vi "getClassInfo.vi"(0 "reference":refnum<class "ClassNode.lvclass">, 5 "error in (no error)":errorcluster) -> (9 "ClassPathUnmodified":path, 11 "methods(string)":string, 12 "Base class.bounds":T1 {"height" format="%.2f"; "width" format="%.2f"; "y" format="%.2f"; "x" format="%.2f"}, 13 "attributes(string)":string, 14 "reference out":refnum<class "ClassNode.lvclass">, 15 "className":string, 16 "attributes":string[](array[string]), 17 "methods":string[](array[string]), 18 "ClassPath":path, 19 "error out":errorcluster)   [LabVIEW 2012, in "ClassNode.lvclass"]
uses:
  <resource>/Framework/Providers/Open_GDS/UML/ClassNode_class/ClassNode.lvclass
  <resource>/Framework/Providers/Open_GDS/UML/General/Rectangle/Rectangle Rectangle2D.ctl
  <resource>/Framework/Providers/Open_GDS/UML/MultiLineString_class/MultiLineString.lvclass
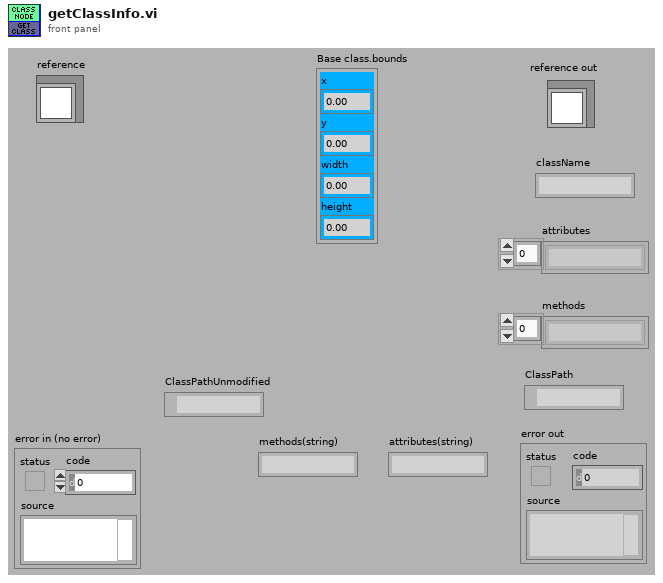
[diagram p1: front panel]
types:
  T1 = typedef "Rectangle Rectangle2D.ctl" = cluster{"x":dbl, "y":dbl, "width":dbl, "height":dbl}
  T2 = typedef "ClassNode.lvclass/ObjectAttributes.ctl" = cluster{"Base class":T3, "midHeight":dbl, "botHeight":dbl, "name":refnum<class "MultiLineString.lvclass">, "attributes":refnum<class "MultiLineString.lvclass">, "methods":refnum<class "MultiLineString.lvclass">, "DEFAULT_COMPARTMENT_HEIGHT":i32, "DEFAULT_WIDTH":i32, "DEFAULT_HEIGHT":i32, "showMethods":bool, "showAttributes":bool, "ClassPath":path}
  T3 = typedef "RectangularNode.lvclass/ObjectAttributes.ctl" = cluster{"Base class":T4, "bounds":T1}
  T4 = typedef "AbstractNode.lvclass/ObjectAttributes.ctl" = cluster{"parent":refnum<class "AbstractNode.lvclass">, "children":refnum<class "AbstractNode.lvclass">[], "Hidden":bool}
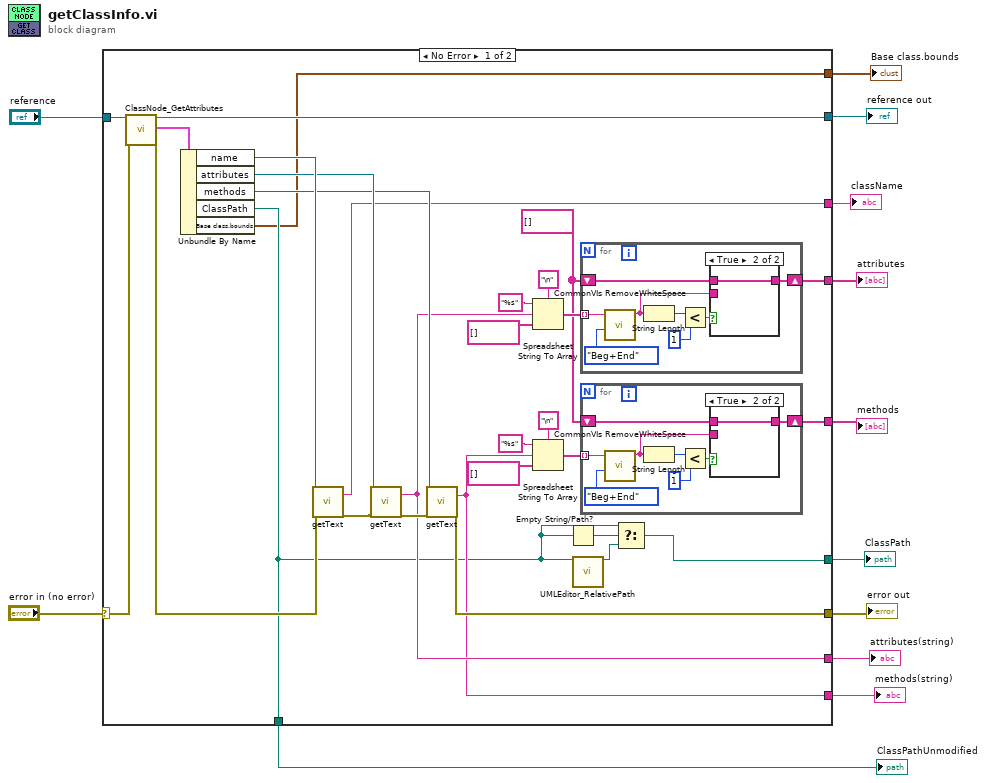
[diagram p0: block diagram]
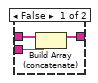
[diagram p2: hidden frame]
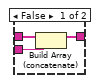
[diagram p3: hidden frame]
diagram:
  n1 = case shown="No Error" "error in (no error)" {
    selector: "error in (no error)" -> [w42 w67]
    tunnel: "reference" -> [w41 w68]
    tunnel: [w35 w67] -> w10
    tunnel: [w39 w68] -> w9
    tunnel: [w31 _] -> w8
    tunnel: [w26 _] -> w7
    tunnel: [w21 _] -> w6
    tunnel: [w14 _] -> w5
    tunnel: [w19 _] -> w4
    tunnel: [w18 _] -> w3
    tunnel: [w16 _] -> w2
    tunnel: [w13 _] -> w1
    frame No Error {
      w20 = string[] []
      n2 = call <resource>:"ClassNode_GetAttributes.vi"("reference in"=w41, "error in (no error)"=w42) -> ("reference out"=w39:refnum<class "ClassNode.lvclass">, "Attributes"=w40:T2, "error out"=w38:errorcluster)  [unwired: 15 out]
      n3 = Unbundle By Name(w40) -> ("name"=w34:refnum<class "MultiLineString.lvclass">, "attributes"=w33:refnum<class "MultiLineString.lvclass">, "methods"=w32:refnum<class "MultiLineString.lvclass">, "ClassPath"=w16:path, "Base class.bounds"=w13:T1)
      n4 = call-dynamic "getText.vi"("reference"=w34, "error in (no error)"=w38) -> ("text"=w31:string, "error out"=w37:errorcluster)  [unwired: 16 out]
      n5 = call-dynamic "getText.vi"("reference"=w33, "error in (no error)"=w37) -> ("text"=w19:string, "error out"=w36:errorcluster)  [unwired: 16 out]
      n6 = call-dynamic "getText.vi"("reference"=w32, "error in (no error)"=w36) -> ("text"=w18:string, "error out"=w35:errorcluster)  [unwired: 16 out]
      n7 = Spreadsheet String To Array(delimiter (Tab)="\n", format string="%s", spreadsheet string=w19, array type (2D Dbl)=string[] []) -> (array=w27:string[])
      n8 = Spreadsheet String To Array(delimiter (Tab)="\n", format string="%s", spreadsheet string=w18, array type (2D Dbl)=string[] []) -> (array=w25:string[])
      n9 = Empty String/Path?(string/path=w16) -> (empty?=w17:bool)
      n10 = call <resource>:"UMLEditor_RelativePath.vi"("Path In"=w16) -> ("ConvertToAbsolutePath(If possible)"=w15:path)  [unwired: 1 in, 17 out]
      n11 = for {
        tunnel: w27 -> [w62] mode=indexing
        shift-right: [w55] -> w26
        shift-left: w20 -> [w57]
        n12 = call <resource>:"CommonVIs RemoveWhiteSpace.vi"("Remove from"=enum16{"Begining", "End", "Beg+End", "All"}."Beg+End", "String in"=w62) -> ("String out"=w56:string)  [unwired: 2 in, 3 out]
        n13 = String Length(string=w56) -> (length=w60:i32)
        n14 = Less?(x=w60, y=1) -> (x < y?=w58:bool)
        n15 = case shown="True" w58 {
          tunnel: w57 -> [w65 w66]
          tunnel: w56 -> [w64 _]
          tunnel: [w63 w66] -> w55
          frame False {
            n16 = Build Array (concatenate)(w65, w64) -> (w63:string[])
          }
          frame True {
          }
        }
      }
      n17 = for {
        tunnel: w25 -> [w50] mode=indexing
        shift-right: [w43] -> w21
        shift-left: w20 -> [w45]
        n18 = call <resource>:"CommonVIs RemoveWhiteSpace.vi"("Remove from"=enum16{"Begining", "End", "Beg+End", "All"}."Beg+End", "String in"=w50) -> ("String out"=w44:string)  [unwired: 2 in, 3 out]
        n19 = String Length(string=w44) -> (length=w48:i32)
        n20 = Less?(x=w48, y=1) -> (x < y?=w46:bool)
        n21 = case shown="True" w46 {
          tunnel: w45 -> [w53 w54]
          tunnel: w44 -> [w52 _]
          tunnel: [w51 w54] -> w43
          frame False {
            n22 = Build Array (concatenate)(w53, w52) -> (w51:string[])
          }
          frame True {
          }
        }
      }
      n23 = Select(t=w16, s=w17, f=w15) -> (s? t:f=w14:path)
    }
    frame Error {
    }
  }
  "reference out" <- w9
  "error out" <- w10
  "className" <- w8
  "attributes" <- w7
  "methods" <- w6
  "ClassPath" <- w5
  "attributes(string)" <- w4
  "methods(string)" <- w3
  "ClassPathUnmodified" <- w2
  "Base class.bounds" <- w1
